vi "Check Read Succeeded.vi"(8 "error in (no error)":errorcluster, 11 "Profile Rsp":T1) -> (0 "error out":errorcluster, 3 "Succeeded?":bool)   [LabVIEW 2014]
uses:
  Public/Clusters/Read Batch Profile Rsp.ctl
  Keyence LJ-V7000.lvlib
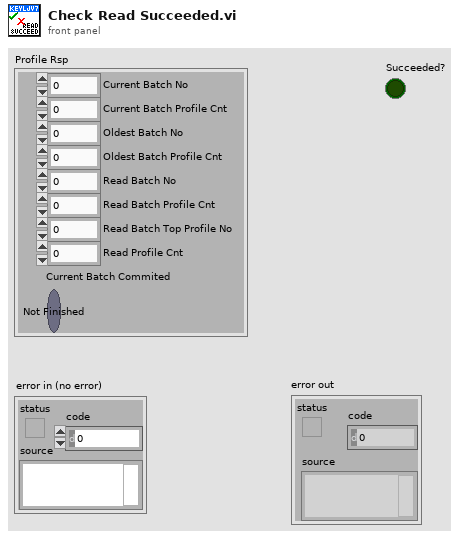
[diagram p1: front panel]
types:
  T1 = typedef "Keyence LJ-V7000.lvlib/Read Batch Profile Rsp.ctl" = cluster{"Current Batch No":u32, "Current Batch Profile Cnt":u32, "Oldest Batch No":u32, "Oldest Batch Profile Cnt":u32, "Read Batch No":u32, "Read Batch Profile Cnt":u32, "Read Batch Top Profile No":u32, "Read Profile Cnt":u8, "Current Batch Commited":bool}
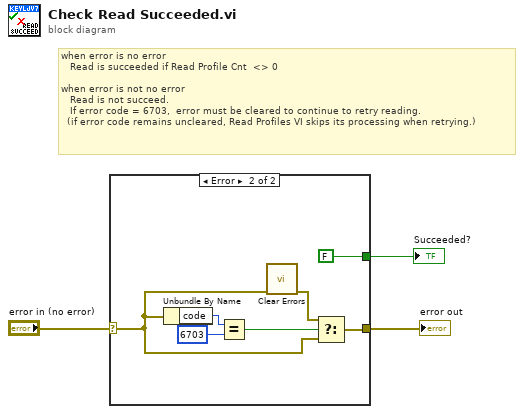
[diagram p0: block diagram]
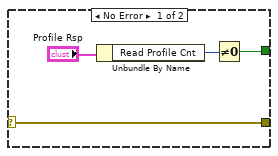
[diagram p2: hidden frame]
diagram:
  # "when error is no error\n   Read is succeeded if Read Profile Cnt  <> 0\n\nwhen error is not no error\n   Read is not succeed.\n   If error code = 6703,  error must be cleared to continue to retry reading.\n  (if error code remains uncleared, Read Profiles VI skips its processing when retrying.)"
  n1 = case shown="Error" "error in (no error)" {
    selector: "error in (no error)" -> [w4 w9]
    tunnel: [w5 FALSE] -> w2
    tunnel: [w4 w8] -> w1
    frame No Error {
      n2 = Unbundle By Name("Profile Rsp") -> ("Read Profile Cnt"=w6:u8)
      n3 = Not Equal To 0?(x=w6) -> (x != 0?=w5:bool)
    }
    frame Error {
      n4 = Unbundle By Name(w9) -> ("code"=w14:i32)
      n5 = Equal?(x=w14, y=6703) -> (x = y?=w11:bool)
      n6 = call <vilib>:"Clear Errors.vi"("error in (no error)"=w9) -> ("error out"=w10:errorcluster)  [unwired: 5 in, 1 out]
      n7 = Select(t=w10, s=w11, f=w9) -> (s? t:f=w8:errorcluster)
    }
  }
  "error out" <- w1
  "Succeeded?" <- w2
